vi "DS402 Drive - Get Slave IOVars.vi"(8 "error in (no error)":errorcluster, 9 "SW Index":i32, 10 "CW Index":i32, 11 "ECAT Slave in":refnum<k21>="ni.var.io://localhost/EtherCAT Master/Device") -> (0 "error IO":errorcluster, 1 "DS402 IOV":T1, 2 "ECAT IO Variables":refnum<k21>[](array[refnum]), 3 "ECAT Slave out":refnum<k21>="ni.var.io:/", 4 "Modules":refnum<k21>[](array[refnum]))   [LabVIEW 2016, in "Scan Engine Custom Device.lvlib"]
uses:
  Scan Engine Custom Device.lvlib
  Type Defs/DS402 Drive ECAT Slave Action IOV Cluster.ctl
  DS402 StateMachine/Library/controls/state.ctl
  <resource>/objmgr/IndComECAT.rc
  <vilib>/NI Veristand/Custom Device Tools/Custom Device Utility Library/Custom Device Utility Library.lvlib
  DS402 StateMachine/Library/DS402.lvlib
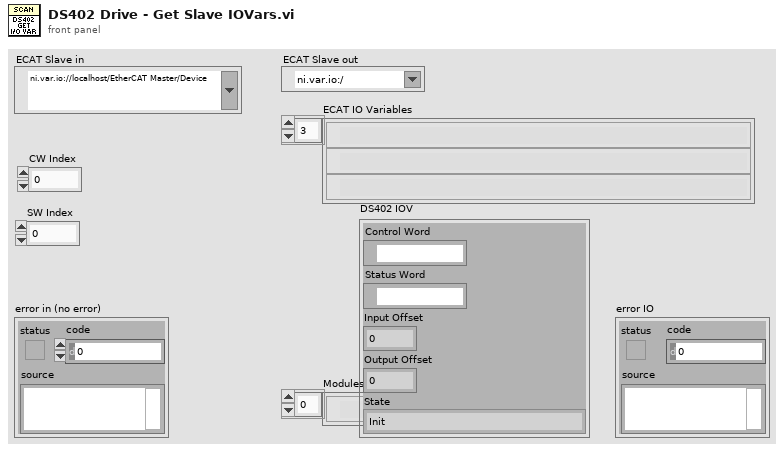
[diagram p1: front panel]
types:
  T1 = typedef "Scan Engine Custom Device.lvlib/DS402 Drive ECAT Slave Action IOV Cluster.ctl" = cluster{"Control Word":refnum<k21>, "Status Word":refnum<k21>, "Input Offset":i32, "Output Offset":i32, "State":T2}
  T2 = typedef "Scan Engine Custom Device.lvlib/DS402.lvlib/state.ctl" = enum16{"Init", "Not Ready to Switch On", "Read Status Word", "Switch on disabled", "Ready to switch on", "Switched on", "Operation enabled", "Fault", "Fault reaction active", "Quick stop active", "Shutdown - Bad State", "Shutdown - Error", "Shutdown - Normal", "Shutdown - Fault"}
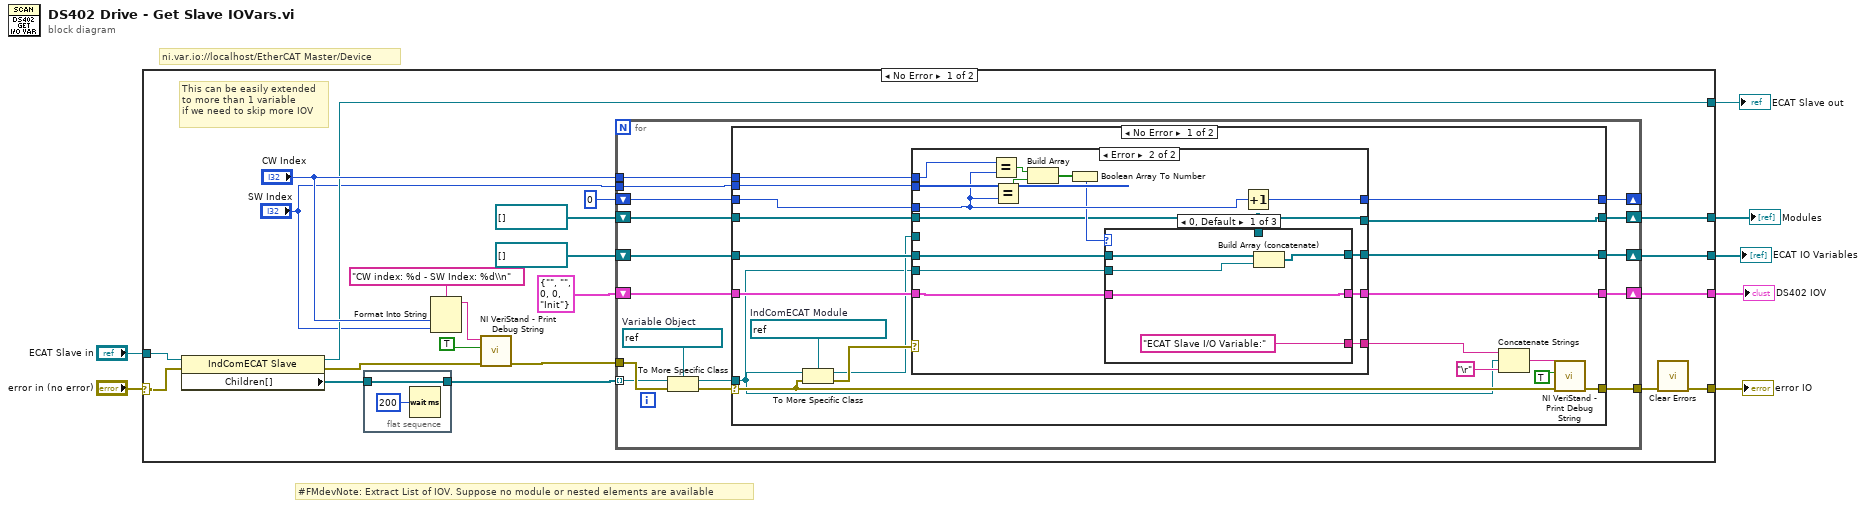
[diagram p0: block diagram]
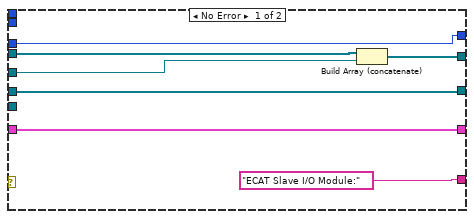
[diagram p2: hidden frame]
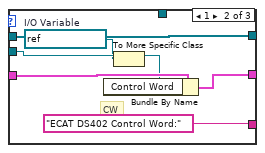
[diagram p3: hidden frame]
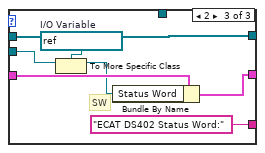
[diagram p4: hidden frame]
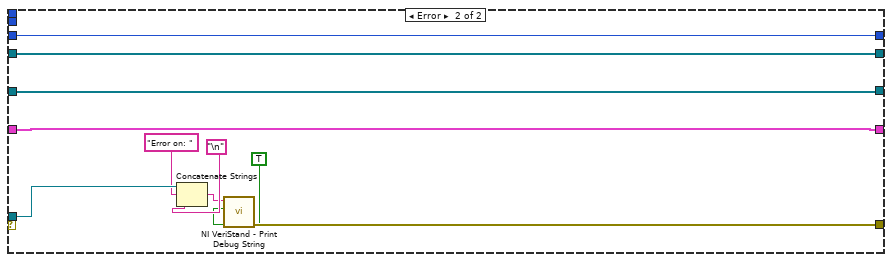
[diagram p5: hidden frame]
diagram:
  # "#FMdevNote: Extract List of IOV. Suppose no module or nested elements are available"
  # "ni.var.io://localhost/EtherCAT Master/Device"
  n1 = case shown="No Error" "error in (no error)" {
    selector: "error in (no error)" -> [w27 w119]
    tunnel: [w19 w119] -> w3
    tunnel: "ECAT Slave in" -> [w28 w118]
    tunnel: [w11 w118] -> w6
    tunnel: [w22 _] -> w4
    tunnel: [w20 _] -> w2
    tunnel: [w16 _] -> w1
    frame No Error {
      # "This can be easily extended\nto more than 1 variable\nif we need to skip more IOV"
      n2 = property class="IndComECAT Slave"(reference=w28, error in=w27) -> (reference out=w11:refnum<k21>, error out=w14:errorcluster, "Children[]"=w25:refnum<k21>[])
      n3 = flat-sequence {
        tunnel: w25 -> [w30]
        tunnel: [w30] -> w24
        frame #0 {
          n4 = Wait (ms)(milliseconds to wait=u32 200) -> ()  [unwired: 1 out]
        }
      }
      n5 = Format Into String(format string="CW index: %d - SW Index: %d\\n", "CW Index", "SW Index") -> (resulting string=w10:string)  [unwired: 2 in, 1 out]
      n6 = call <vilib>:"NI VeriStand - Print Debug String.vi"("error in (no error)"=w14, "Add to log file? (T)"=TRUE, "Message"=w10) -> ("error out"=w13:errorcluster)  [unwired: 8 in]
      n7 = for {
        tunnel: w24 -> [w42] mode=indexing
        tunnel: w13 -> [w46]
        tunnel: [w45] -> w26
        shift-right: [w41] -> w22
        shift-left: refnum<k21>[] [] -> [w40]
        shift-right: [w37] -> w20
        shift-left: refnum<k21>[] [] -> [w38]
        tunnel: "CW Index" -> [w36]
        shift-right: [w34] -> _
        shift-left: 0 -> [w35]
        tunnel: "SW Index" -> [w33]
        shift-right: [w31] -> w16
        shift-left: T1 {"Control Word"="", "Status Word"="", "Input Offset"=0, "Output Offset"=0, "State"=enum."Init"} ("DS402 IOV") -> [w32]
        w39 = refnum<k21> refnum  # Variable Object
        n8 = To More Specific Class(target class=w39, reference=w42, error in=w46) -> (specific class reference=w43:refnum<k21>, error out=w44:errorcluster)
        n9 = case shown="No Error" w44 {
          selector: w44 -> [w50 _]
          tunnel: w43 -> [w47 w116]
          tunnel: [w51 w112] -> w45
          tunnel: [w65 w117] -> w41
          tunnel: w40 -> [w66 w117]
          tunnel: w38 -> [w62 w110]
          tunnel: [w61 w110] -> w37
          tunnel: w36 -> [w60 _]
          tunnel: w35 -> [w59 w109]
          tunnel: [w58 w109] -> w34
          tunnel: w33 -> [w57 _]
          tunnel: w32 -> [w56 w108]
          tunnel: [w55 w108] -> w31
          frame No Error {
            w64 = refnum<k21> refnum  # IndComECAT Module
            n10 = To More Specific Class(target class=w64, reference=w47, error in=w50) -> (specific class reference=w49:refnum<k21>, error out=w63:errorcluster)
            n11 = case shown="Error" w63 {
              tunnel: w66 -> [w71 w88]
              tunnel: [w71 w86] -> w65
              tunnel: w47 -> [_ w87]
              tunnel: w62 -> [w73 w74]
              tunnel: [w72 w74] -> w61
              tunnel: w49 -> [w70 _]
              tunnel: w60 -> [_ w83]
              tunnel: w59 -> [w69 w82]
              tunnel: [w69 w85] -> w58
              tunnel: w57 -> [_ w84]
              tunnel: w56 -> [w68 w77]
              tunnel: [w68 w76] -> w55
              tunnel: ["ECAT Slave I/O Module:" w75] -> w48
              frame No Error {
                n12 = Build Array (concatenate)(w73, w70) -> (w72:refnum<k21>[])
              }
              frame Error {
                n13 = Equal?(x=w83, y=w82) -> (x = y?=w81:bool)
                n14 = Equal?(x=w84, y=w82) -> (x = y?=w80:bool)
                n15 = Build Array(w81, w80) -> (w79:bool[])
                n16 = Boolean Array To Number(Boolean array=w79) -> (number=w78:u32)
                n17 = case shown="0, Default" w78 {
                  tunnel: w88 -> [w93 w100 w105]
                  tunnel: w87 -> [w92 w95 w103]
                  tunnel: [w91 w100 w105] -> w86
                  tunnel: w77 -> [w90 w99 w107]
                  tunnel: [w90 w98 w106] -> w76
                  tunnel: ["ECAT Slave I/O Variable:" "ECAT DS402 Control Word:" "ECAT DS402 Status Word:"] -> w75
                  tunnel: w74 -> [_ _ _]
                  frame 0, Default {
                    n18 = Build Array (concatenate)(w93, w92) -> (w91:refnum<k21>[])
                  }
                  frame 1 {
                    w94 = refnum<k21> refnum  # I/O Variable
                    # "CW"
                    n19 = To More Specific Class(target class=w94, reference=w95) -> (specific class reference=w96:refnum<k21>)  [unwired: 1 in, 1 out]
                    n20 = Bundle By Name(cluster=w99, "Control Word"=w96) -> (w98:T1)
                  }
                  frame 2 {
                    w102 = refnum<k21> refnum  # I/O Variable
                    # "SW"
                    n21 = To More Specific Class(target class=w102, reference=w103) -> (specific class reference=w101:refnum<k21>)  [unwired: 1 in, 1 out]
                    n22 = Bundle By Name(cluster=w107, "Status Word"=w101) -> (w106:T1)
                  }
                }
                n23 = Increment(x=w82) -> (x+1=w85:i32)
              }
            }
            n24 = Concatenate Strings(w48, w47, "\r") -> (w54:string)
            n25 = call <vilib>:"NI VeriStand - Print Debug String.vi"("error in (no error)"=w50, "Add to log file? (T)"=TRUE, "Message"=w54) -> ("error out"=w51:errorcluster)  [unwired: 8 in]
          }
          frame Error {
            n26 = Concatenate Strings(w116, "Error on: ", "\n") -> (w113:string)
            n27 = call <vilib>:"NI VeriStand - Print Debug String.vi"("Add to log file? (T)"=TRUE, "Message"=w113) -> ("error out"=w112:errorcluster)  [unwired: 9 in]
          }
        }
      }
      n28 = call <vilib>:"Clear Errors.vi"("error in (no error)"=w26) -> ("error out"=w19:errorcluster)  [unwired: 5 in, 1 out]
    }
    frame Error {
    }
  }
  "error IO" <- w3
  "ECAT Slave out" <- w6
  "ECAT IO Variables" <- w4
  "Modules" <- w2
  "DS402 IOV" <- w1
